vi "Create Status Log Folder.vi"(7 "QRD":T1, 8 "error in":errorcluster) -> (0 "error out":errorcluster, 5 "QRD Out":T1)   [LabVIEW 2025]
uses:
  Controls/Queues-Refs-Data.ctl
  Builds/Queue Wrappers.lvlibp/Q Packet.ctl
  Builds/Queue Wrappers.lvlibp
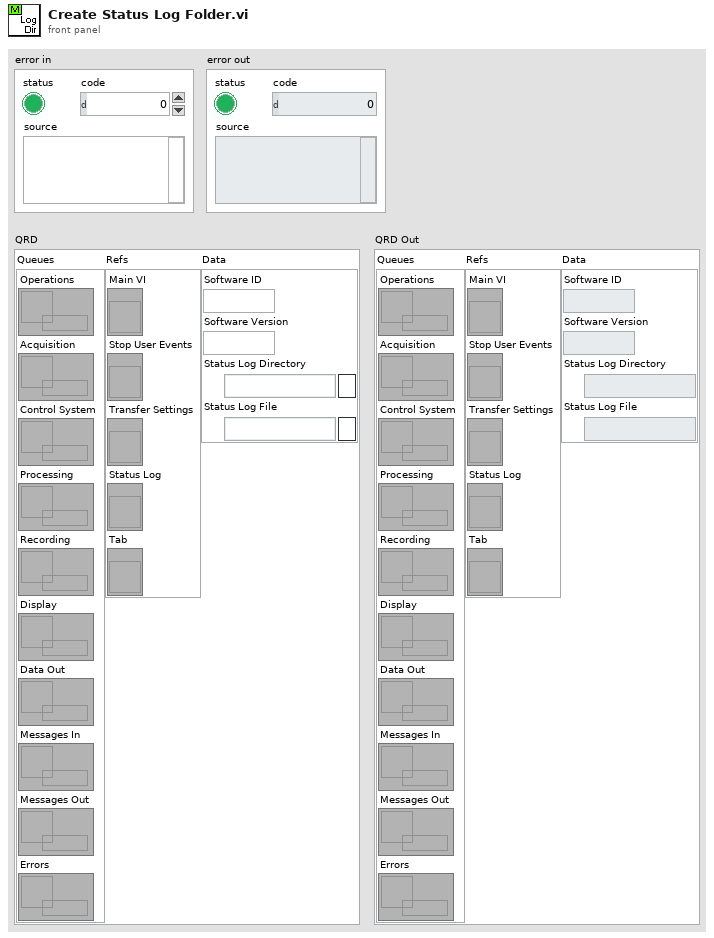
[diagram p1: front panel]
types:
  T1 = typedef "Queues-Refs-Data.ctl" = cluster{"Queues":cluster{"Operations":refnum<queue>, "Acquisition":refnum<queue>, "Control System":refnum<queue>, "Processing":refnum<queue>, "Recording":refnum<queue>, "Display":refnum<queue>, "Data Out":refnum<queue>, "Messages In":refnum<queue>, "Messages Out":refnum<queue>, "Errors":refnum<queue>}, "Refs":cluster{"Main VI":refnum<vi>, "Stop User Events":refnum<vi>, "Transfer Settings":refnum<vi>, "Status Log":refnum<vi>, "Tab":refnum<vi>}, "Data":cluster{"Software ID":string, "Software Version":string, "Status Log Directory":path, "Status Log File":path}}
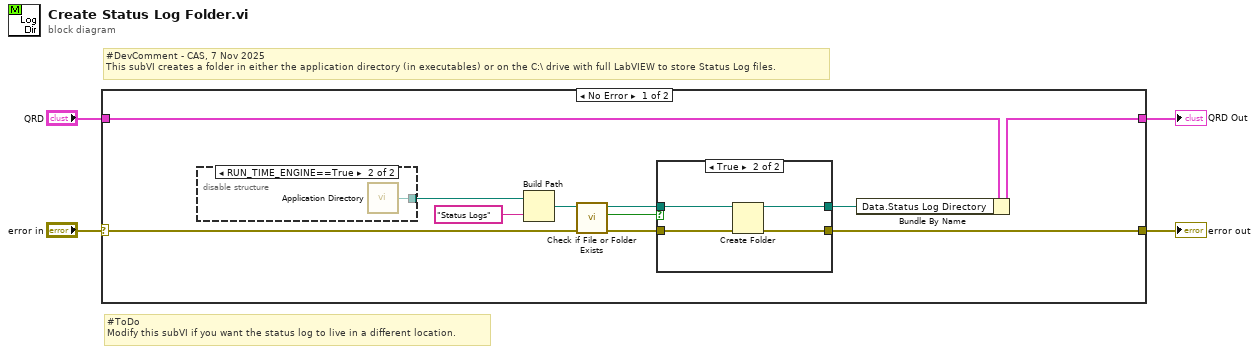
[diagram p0: block diagram]
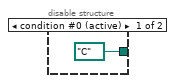
[diagram p2: hidden frame]
diagram:
  # "#ToDo\nModify this subVI if you want the status log to live in a different location."
  # "#DevComment - CAS, 7 Nov 2025\nThis subVI creates a folder in either the application directory (in executables) or on the C:\\ drive with full LabVIEW to store Status Log files."
  n1 = case shown="No Error" "error in" {
    selector: "error in" -> [w14 w25]
    tunnel: [w8 w25] -> w3
    tunnel: "QRD" -> [w7 w24]
    tunnel: [w5 w24] -> w1
    frame No Error {
      n2 = disable-structure shown="RUN_TIME_ENGINE==True" {
        disable-tunnel: [path "C:/" ("path") w17] -> w9
        frame condition #0 (active) {
        }
        frame condition #1 {
          n3 = call <vilib>:"Application Directory.vi"() -> ("Application Directory"=w17:path)
        }
      }
      n4 = Build Path(base path=w9, name or relative path="Status Logs") -> (appended path=w10:path)
      n5 = call <vilib>:"Check if File or Folder Exists.vi"("error in (no error)"=w14, "path"=w10) -> ("error out"=w13:errorcluster, "file or folder exists?"=w11:bool, "dup path"=w12:path)  [unwired: 7 in]
      n6 = case shown="True" w11 {
        tunnel: w13 -> [w18 w23]
        tunnel: w12 -> [w19 w22]
        tunnel: [w19 w21] -> w6
        tunnel: [w18 w20] -> w8
        frame False {
        }
        frame True {
          n7 = Create Folder(path (use dialog)=w22, error in=w23) -> (created path=w21:path, error out=w20:errorcluster)  [unwired: 1 in, 1 out]
        }
      }
      n8 = Bundle By Name(cluster=w7, "Data.Status Log Directory"=w6) -> (w5:T1)
    }
    frame Error {
    }
  }
  "error out" <- w3
  "QRD Out" <- w1
